vi "Position Lat lon Indicator.vi"(8 "error in (no error)":errorcluster, 9 "Mission Methods":refnum<vi>, 10 "Longitude":refnum<vi>, 11 "Latitude":refnum<vi>) -> (0 "error out":errorcluster)   [LabVIEW 2014]
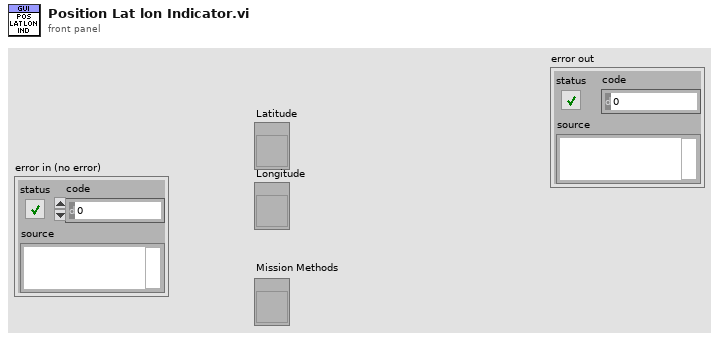
[diagram p1: front panel]
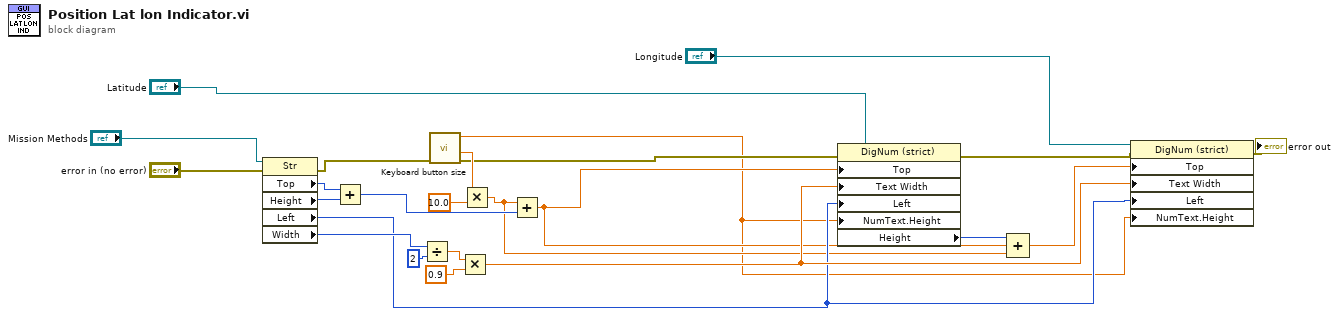
[diagram p0: block diagram]
diagram:
  n1 = property class="Str"(reference="Mission Methods", error in="error in (no error)") -> (error out=w20:errorcluster, "Top"=w22:i32, "Height"=w21:u32, "Left"=w6:i32, "Width"=w9:u32)  [unwired: 1 out]
  n2 = Add(x=w22, y=w21) -> (x+y=w19:u32)
  n3 = Divide(x=w9, y=u32 2) -> (x/y=w8:dbl)
  n4 = call "Keyboard button size.vi"("error in (no error)"=w20) -> ("error out"=w13:errorcluster, "Key Spacing"=w18:dbl, "Key Height"=w1:dbl)  [unwired: 7 in, 1 out]
  n5 = Multiply(x=w8, y=0.9) -> (x*y=w7:dbl)
  n6 = Multiply(x=w18, y=10.0) -> (x*y=w4:dbl)
  n7 = Add(x=w4, y=w19) -> (x+y=w5:dbl)
  n8 = property class="DigNum (strict)"(reference="Latitude", error in=w13, "Top"=w5, "Text Width"=w7, "Left"=w6, "NumText.Height"=w1) -> (error out=w12:errorcluster, "Height"=w2:u32)  [unwired: 1 out]
  n9 = Compound Arithmetic op=ADD(w2, w5, w4) -> (w3:dbl)
  n10 = property class="DigNum (strict)"(reference="Longitude", error in=w12, "Top"=w3, "Text Width"=w7, "Left"=w6, "NumText.Height"=w1) -> (error out=→"error out":errorcluster)  [unwired: 1 out]
